vi "Normalize Magnitude.vi"(8 "D":dbl, 9 "C":dbl, 10 "B":dbl, 11 "A":dbl) -> (0 "D'":dbl, 1 "C'":dbl, 2 "B'":dbl, 3 "A'":dbl)   [LabVIEW 2017]
panel:
  # "Normalize Magnitude Teleop Control\nFRC Team 34"
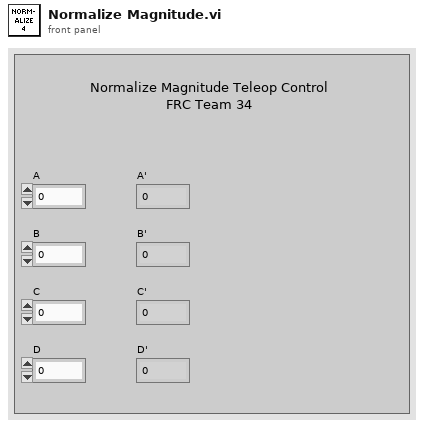
[diagram p1: front panel]
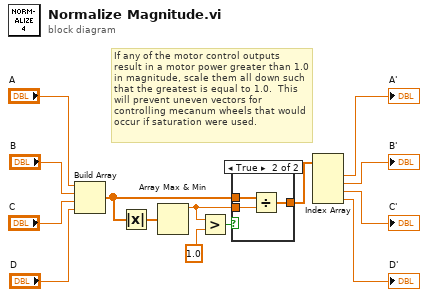
[diagram p0: block diagram]
diagram:
  # "If any of the motor control outputs result in a motor power greater than 1.0 in magnitude, scale them all down such that the greatest is equal to 1.0.  This will prevent uneven vectors for controlling mecanum wheels that would occur if saturation were used."
  n1 = Build Array("A", "B", "C", "D") -> (w4:dbl[])
  n2 = Absolute Value(x=w4) -> (abs(x)=w10:dbl[])
  n3 = Array Max & Min(array=w10) -> (max value=w2:dbl)  [unwired: 3 out]
  n4 = Greater?(x=w2, y=1.0) -> (0:w3:bool)
  n5 = case shown="True" w3 {
    tunnel: w2 -> [_ w18]
    tunnel: [w15 w17] -> w9
    tunnel: w4 -> [w15 w16]
    frame False {
    }
    frame True {
      n6 = Divide(x=w16, y=w18) -> (x/y=w17:dbl[])
    }
  }
  n7 = Index Array(array=w9) -> (element #1=→"A'":dbl, element #2=→"B'":dbl, element #3=→"C'":dbl, element #4=→"D'":dbl)  [unwired: 4 in]
